vi "PresConversion.vi"(11 "A/AI0 (Pin 3)":dbl) -> (3 "Numeric":dbl)   [LabVIEW 2019]
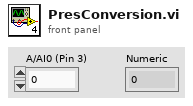
[diagram p1: front panel]
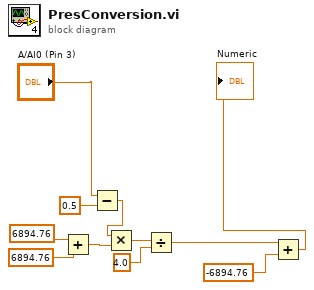
[diagram p0: block diagram]
diagram:
  n1 = Add(x=6894.76, y=6894.76) -> (x+y=w7:dbl)
  n2 = Subtract(x="A/AI0 (Pin 3)", y=0.5) -> (x-y=w4:dbl)
  n3 = Multiply(x=w4, y=w7) -> (x*y=w8:dbl)
  n4 = Divide(x=w8, y=4.0) -> (x/y=w1:dbl)
  n5 = Add(x=w1, y=-6894.76 ("x")) -> (x+y=→"Numeric":dbl)
